vi "SENS_FOM_STAT.vi"(0 "VISA IN":refnum<visa-resource-name>, 1 "FOM ON/OFF":bool, 5 "error in":errorcluster, 7 "Channel":i32) -> (14 "VISA Out":refnum<visa-resource-name>, 19 "error out":errorcluster)   [LabVIEW 2018, in "PNA-X.lvlib"]
doc: "SENSe<cnum>:FOM[:STATe] <bool> \n1735\n\n(Read-Write) Turns Frequency Offset ON and OFF. Frequency offset settings are not enabled until this setting is \nON. \nSend this command (FOM ON) AFTER sending other FOM settings to avoid 'out-or-range' errors. \nParameters \n<cnum> Any existing channel number; if unspecified, value is set to 1. \n<bool> ON (or 1) - turns FOM ON. \nOFF (or 0) - turns FOM OFF. \nExamples SENS:FOM 1 \nsense2:fom:state on \nQuery Syntax SENSe<cnum>:FOM:STATe? \nReturn Type Boolean \nDefault OFF"
uses:
  PNA-X.lvlib
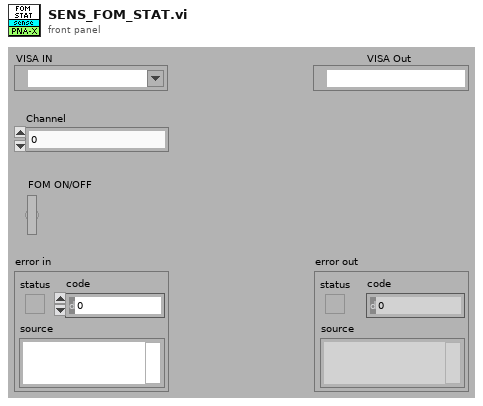
[diagram p1: front panel]
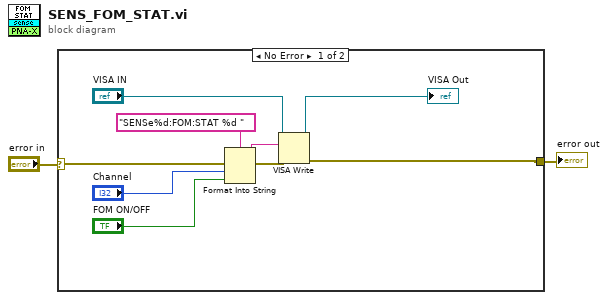
[diagram p0: block diagram]
diagram:
  n1 = case shown="No Error" "error in" {
    selector: "error in" -> [w11 w12]
    tunnel: [w6 w12] -> w1
    frame No Error {
      n2 = Format Into String(format string="SENSe%d:FOM:STAT %d " ("Cmdline"), error in=w11, "Channel", "FOM ON/OFF") -> (resulting string=w9:string, error out=w10:errorcluster)  [unwired: 1 in]
      n3 = VISA Write(VISA resource name="VISA IN", write buffer=w9, error in (no error)=w10) -> (VISA resource name out=→"VISA Out":refnum<visa-resource-name>, error out=w6:errorcluster)  [unwired: 1 out]
    }
    frame Error {
    }
  }
  "error out" <- w1
